vi "Ejercicio 5.vi"() -> (0 "x > y?":bool)   [LabVIEW 2021]
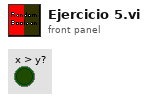
[diagram p1: front panel]
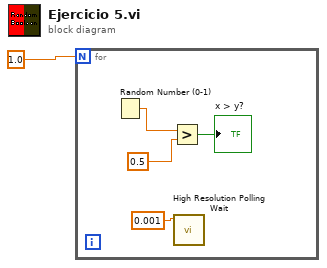
[diagram p0: block diagram]
diagram:
  n1 = for {
    N: 1.0 -> [_]
    n2 = Random Number (0-1)() -> (number: 0 to 1=w3:dbl)
    n3 = Greater?(x=w3, y=0.5) -> (0:→"x > y?":bool)
    n4 = call <vilib>:"High Resolution Polling Wait.vi"("seconds to wait"=0.001) -> ()  [unwired: 10 in, 1 out]
  }
